vi "Offsets Widget Old.vi"(8 "error in (no error)":errorcluster) -> (0 "error out":errorcluster)   [LabVIEW 2013]
uses:
  Popups/Update Offset Actions.ctl
  lib/Data Access Objects/Metadata/Persistant DAO Actions.ctl
  lib/Data Access Objects/Metadata/DAO Actions.ctl
  lib/Global Data/Dataset Source.ctl
  lib/Global Data/Transactions/Dataset Type.ctl
  lib/Apps/Yes No Button.ctl
  lib/Global Data/Transactions/Dataset Transaction Id.ctl
  lib/Data Access Objects/Metadata/DAO Actions with Remove.ctl
  lib/Launcher/Launcher Actions.ctl
  lib/Launcher/NoPanelAppTypes.ctl
  lib/Offsets/Offset Types.ctl
  Popups/Offset Message.ctl
  <vilib>/Utility/miscctls.llb/LVPointTypeDef.ctl
  lib/Data Display/External Sensor Name Offset & Value.ctl
  lib/Offsets Widget/Offset Widget Actions.ctl
  lib/MixedMode/Messages/MM Widget Parameter Changes.ctl
  lib/Apps/GUI Control.ctl
  Popups/Offset Table Component.ctl
  lib/Offsets Widget/Cartesian Or Actuator.ctl
panel:
  in  "HasBeenModified":bool
  in  "External Sensors Label":string[](array[string])
  in  "External Sensors Table":T1[](array[typedef])
  in  "Table 5":T2 {"Table Data 1" format="%^#_7e"}
  in  "Table 4":T2 {"Table Data 1" format="%^#_7e"}
  in  "Table 3":T2 {"Table Data 1" format="%^#_7e"}
  in  "Table 2":T2 {"Table Data 1" format="%^#_7e"}
  in  "Table 1":T2 {"Table Data 1" format="%^#_7e"}
  in  "Row Labels":string[](array[string])
  in  "Table 0":T2 {"Table Data 1" format="%^#_7e"}
  out "Default Data":dbl[][](array[numeric])
  out "Default Transactions":T3[](array[typedef])
  in  "Coordinate Space":T7 caption="Coord"
  in  "Cartesian Type":bool caption="Coord"
  in  "Force Offset Tag":u16(ring) items=["<None>"]
  in  "Offset Type":T8
  in  "Load":bool
  in  "Number Of Samples":i32
  in  "Sample Interval\n(milliseconds)":dbl
  in  "Offset Widget Actions":T9
  in  "Execute":bool
  in  "Cancel":bool
  in  "Ok":bool
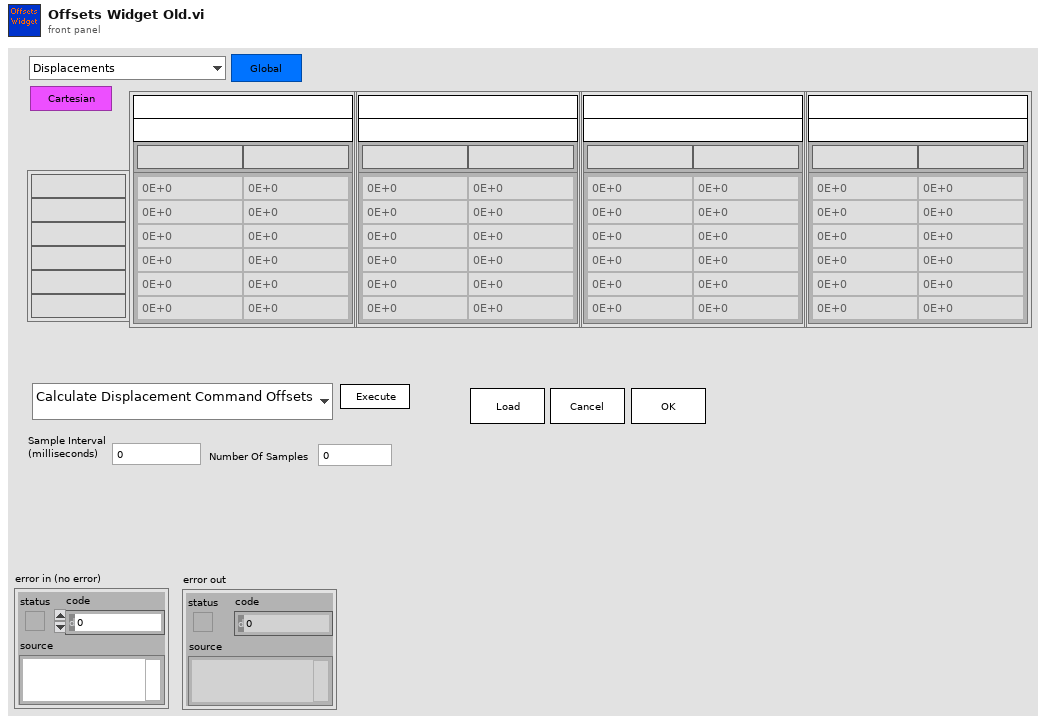
[diagram p1: front panel]
types:
  T1 = typedef "External Sensor Name Offset & Value.ctl" = cluster{"Name":string, "Offset":dbl, "Value 2":dbl}
  T2 = typedef "Offset Table Component.ctl" = cluster{"Table Data 1":dbl[][], "Offset or Current Label":string[], "DOF Label":string, "LBCB Label":string}
  T3 = typedef "Dataset Transaction Id.ctl" = cluster{"Dataset Source":T4, "Dataset Type":T5, "Hold":T6, "Volts":T6, "Tag":string}
  T4 = typedef "Dataset Source.ctl" = enum16{"Continuous", "Hold", "ED", "Volts", "Offsets", "Increments"}
  T5 = typedef "Dataset Type.ctl" = enum16{"LVDT", "Load Cell", "Actuator Command", "Servo Error", "Displacement Command", "Displacement", "Force"}
  T6 = typedef "Yes No Button.ctl" = bool
  T7 = typedef "Cartesian Or Actuator.ctl" = bool
  T8 = typedef "Offset Types.ctl" = enum16{"Displacements", "Forces", "External Sensors"}
  T9 = typedef "Offset Widget Actions.ctl" = enum16{"Calculate Displacement Command Offsets", "Calculate Displacement Offsets", "Calculate Force Offsets", "Calculate External Sensor Offsets"}
  T10 = typedef "GUI Control.ctl" = cluster{"Command":T11, "LBCB Number":enum16{"LBCB1", "LBCB2"}}
  T11 = typedef "MM Widget Parameter Changes.ctl" = enum16{"Start", "Stop All", "Control Enabled", "Control Disabled"}
  T12 = typedef "Offset Message.ctl" = cluster{"Update Offset Actions":T13, "Offset Type":T8, "Coordinate Space":bool, "Cartesian Type":bool}
  T13 = typedef "Update Offset Actions.ctl" = enum16{"Update Table", "Calculate Cartesian Offsets", "Redo Headers", "Has Been Modified", "Exit"}
  T14 = typedef "Persistant DAO Actions.ctl" = enum16{"Init", "Get", "Set", "Load", "Save"}
  T15 = typedef "LVPointTypeDef.ctl" = cluster{"Horizontal":i16, "Vertical":i16}
  T16 = typedef "DAO Actions.ctl" = enum16{"Init", "Get", "Set"}
  T17 = typedef "LVRectTypeDef.ctl" = cluster{"Left":i16, "Top":i16, "Right":i16, "Bottom":i16}
  T18 = typedef "App Parameters.ctl" = cluster{"Monitor Loop":T19, "Ramp Time":T19, "Log Loop":T19, "TCP to DAQ":T19, "Logging Directory":path, "Log File Size (MBytes)":i64, "Volt Logging Loop":T19, "2 LBCB Archiving Mode":bool, "Fake":bool}
  T19 = typedef "Timing Parameters.ctl" = cluster{"Interval":dbl, "Rate ":dbl}
  T20 = typedef "Number Of LBCBs.ctl" = enum16{"1", "2"}
  T21 = cluster{"Table Data 1":dbl[][], "Offset or Current Label":string[], "DOF Label":string, "LBCB Label":string}
  T22 = typedef "DAO Actions with Remove.ctl" = enum16{"Init", "Get", "Set", "Remove"}
  T23 = typedef "NoPanelAppTypes.ctl" = enum16{"NTCP Socket", "Data Archiving", "DAQ Link", "Control Loops", "Cmd Disp Diffs", "LBCB Data", "Limits", "Mixed Mode Widget", "Offsets", "Debug"}
  T24 = typedef "Launcher Actions.ctl" = enum16{"Launch", "Stop All", "Stop", "Kill", "Running?", "Init"}
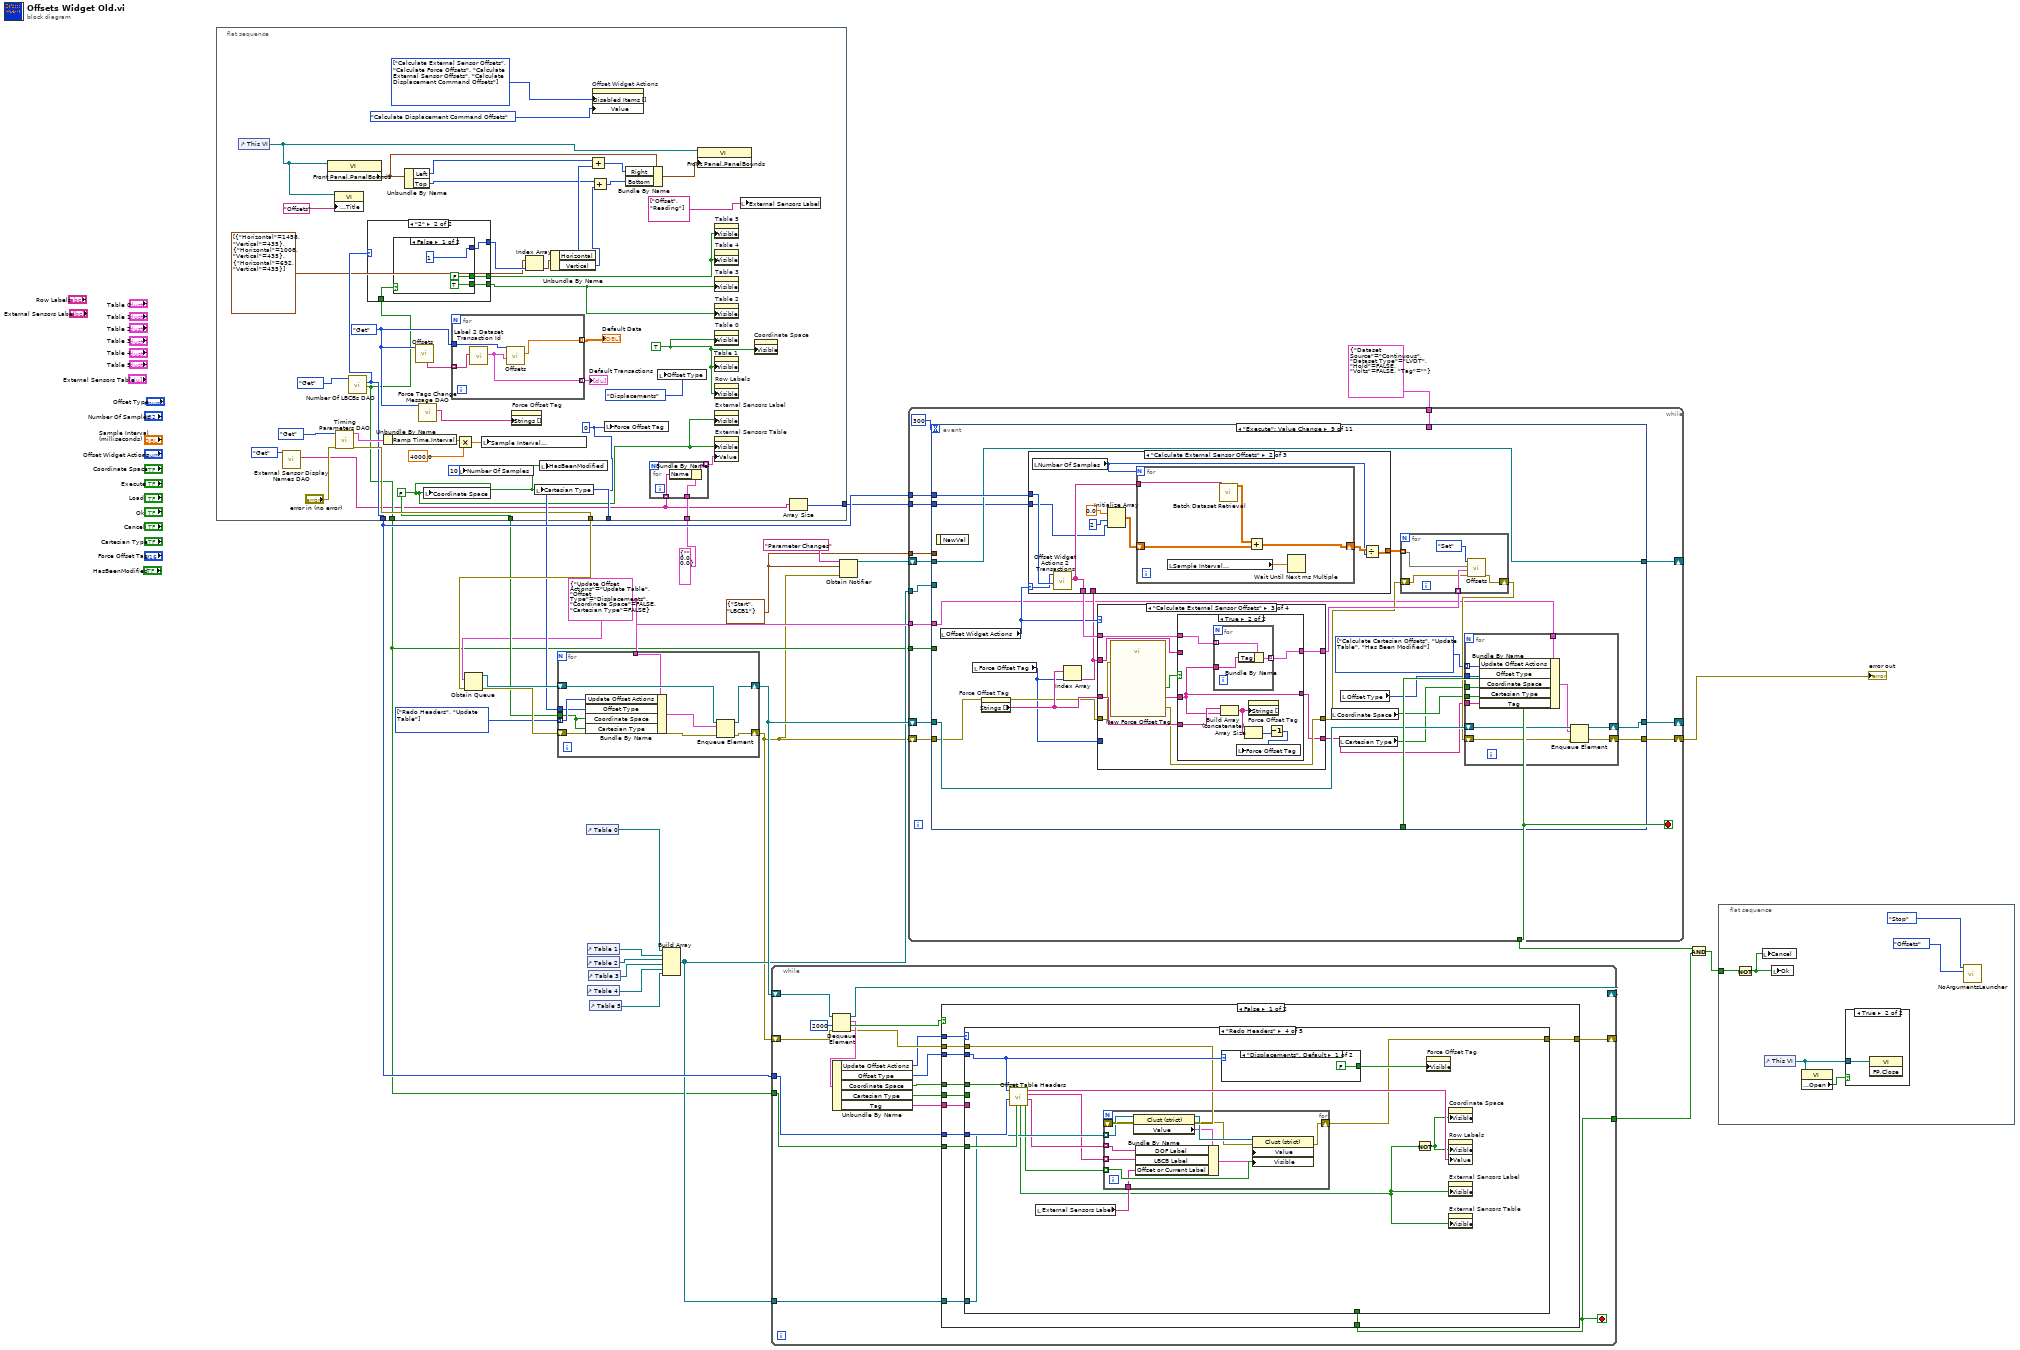
[diagram p0: block diagram]
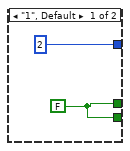
[diagram p2: hidden frame]
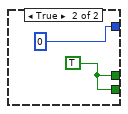
[diagram p3: hidden frame]
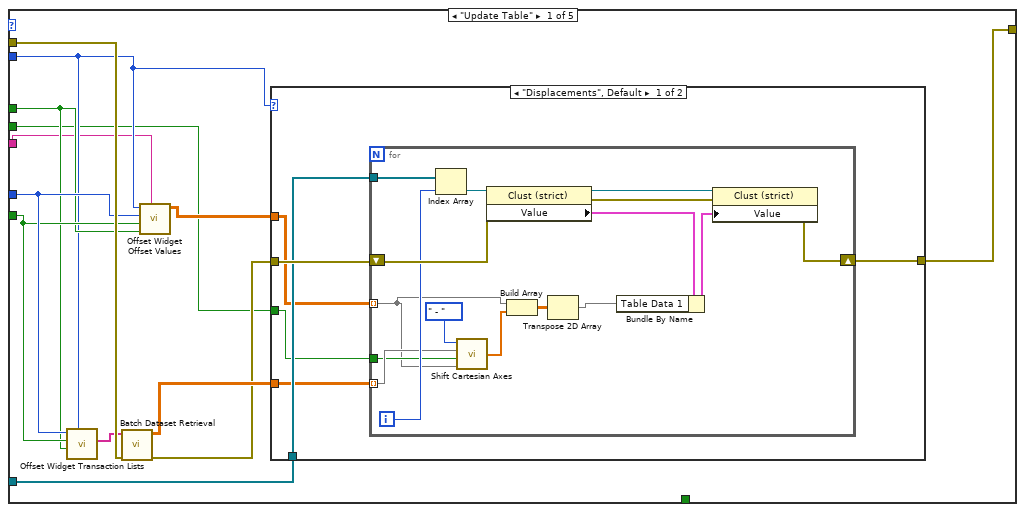
[diagram p5: hidden frame]
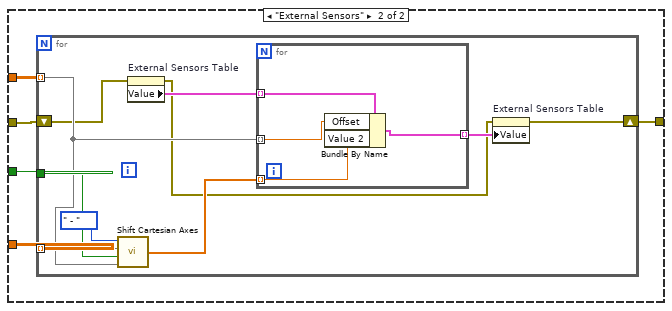
[diagram p6: hidden frame]
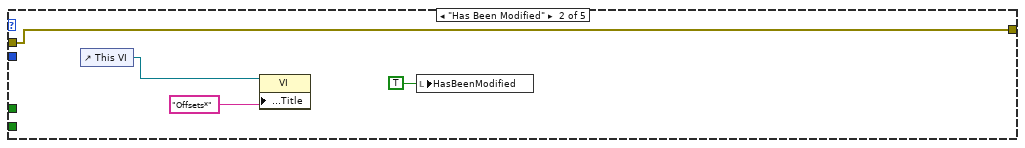
[diagram p7: hidden frame]
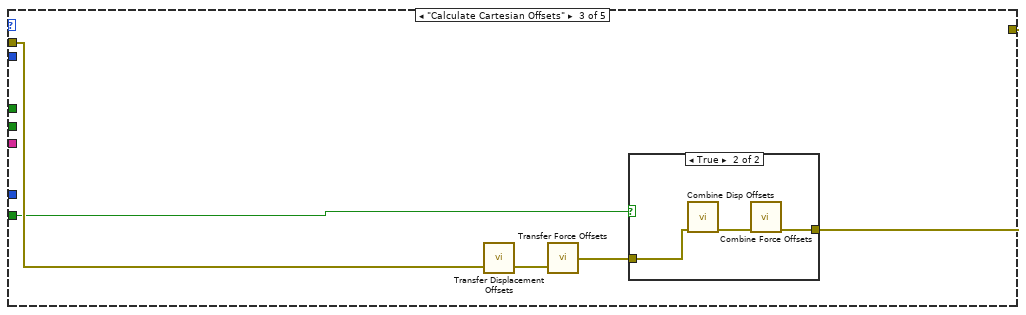
[diagram p8: hidden frame]
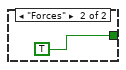
[diagram p10: hidden frame]
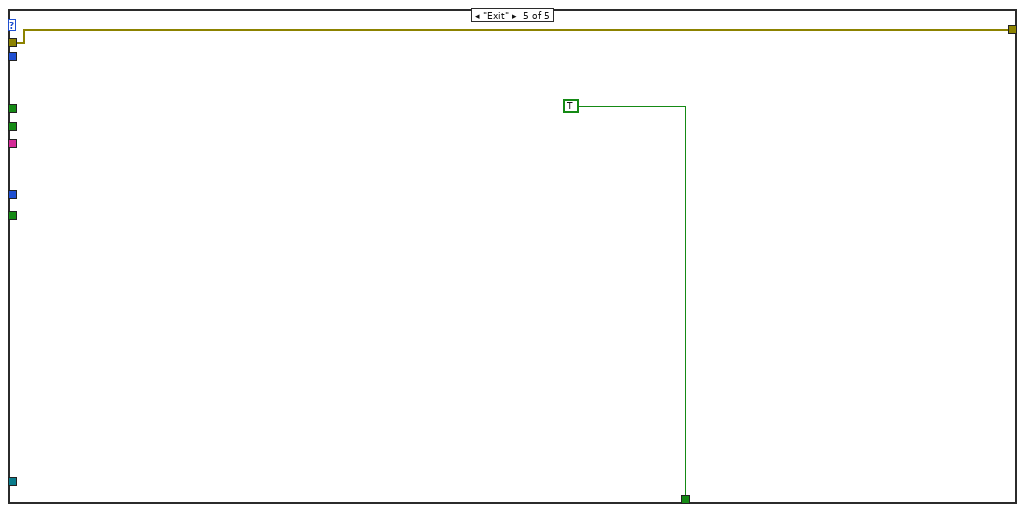
[diagram p11: hidden frame]
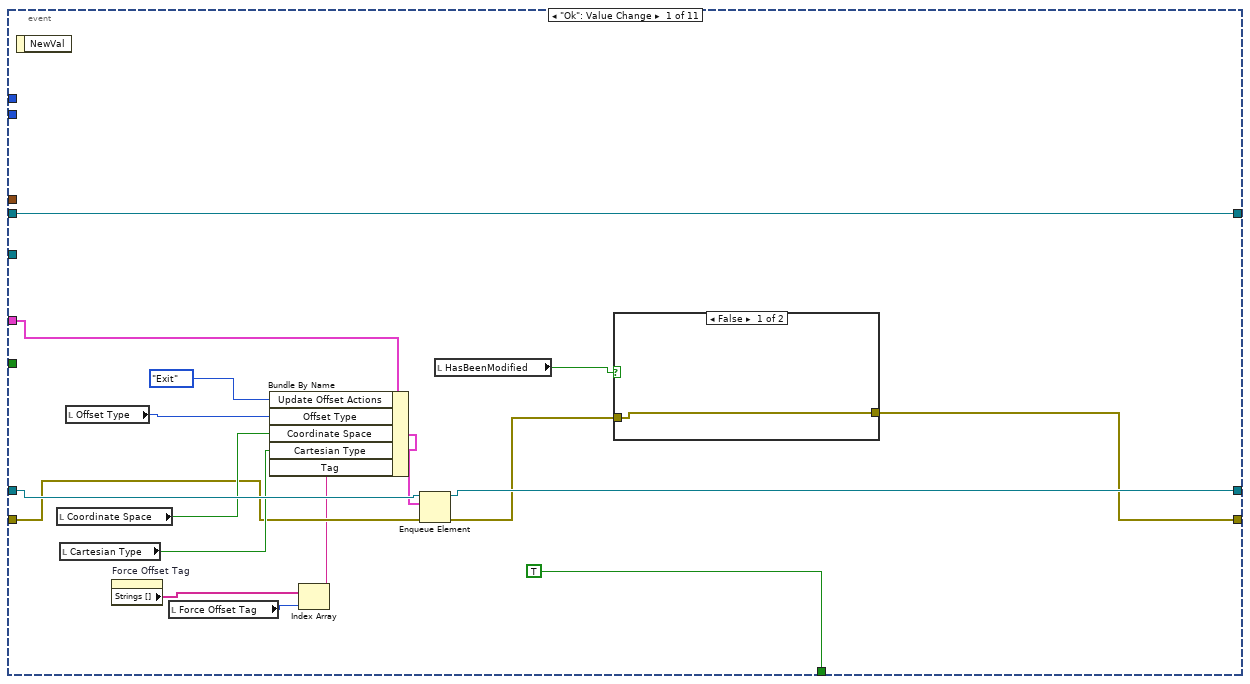
[diagram p13: hidden frame]
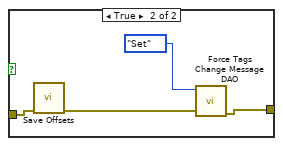
[diagram p14: hidden frame]
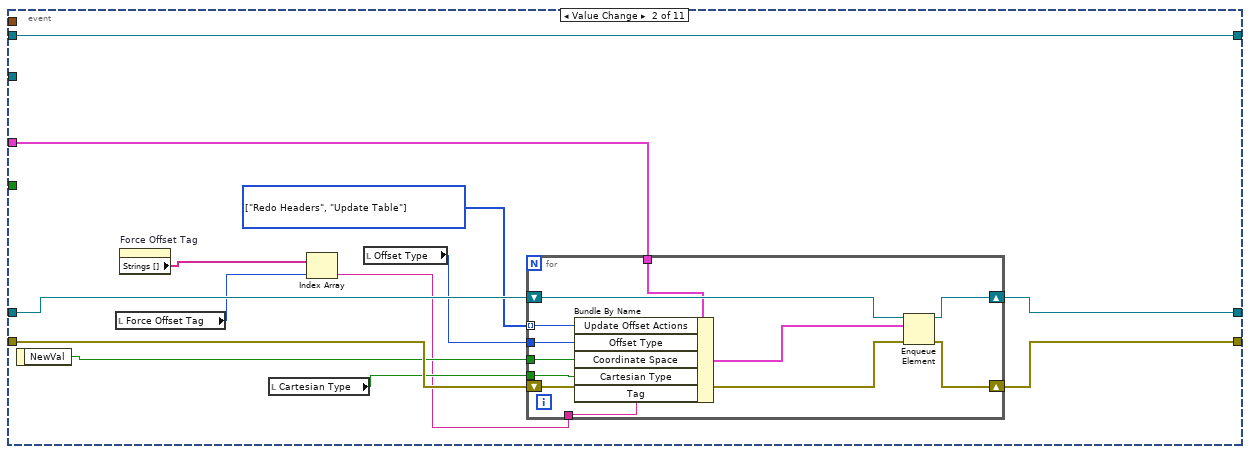
[diagram p15: hidden frame]
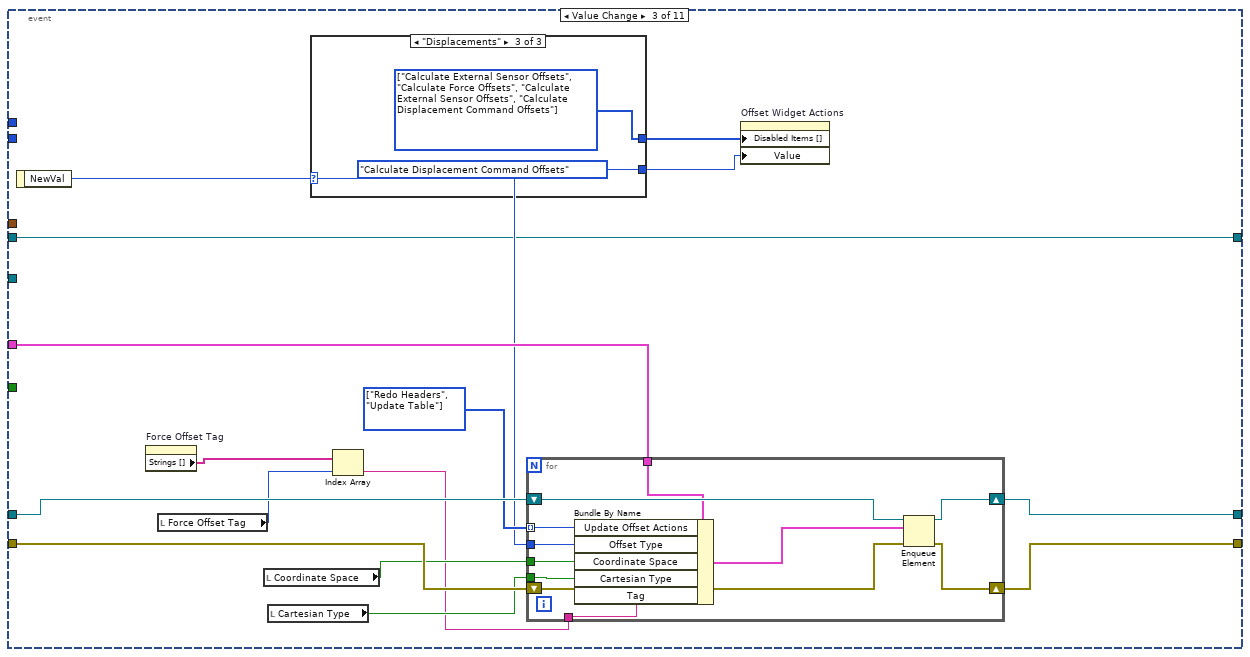
[diagram p16: hidden frame]
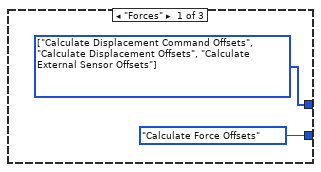
[diagram p17: hidden frame]
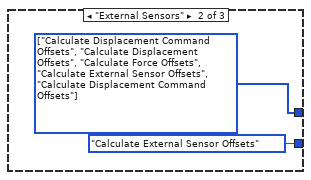
[diagram p18: hidden frame]
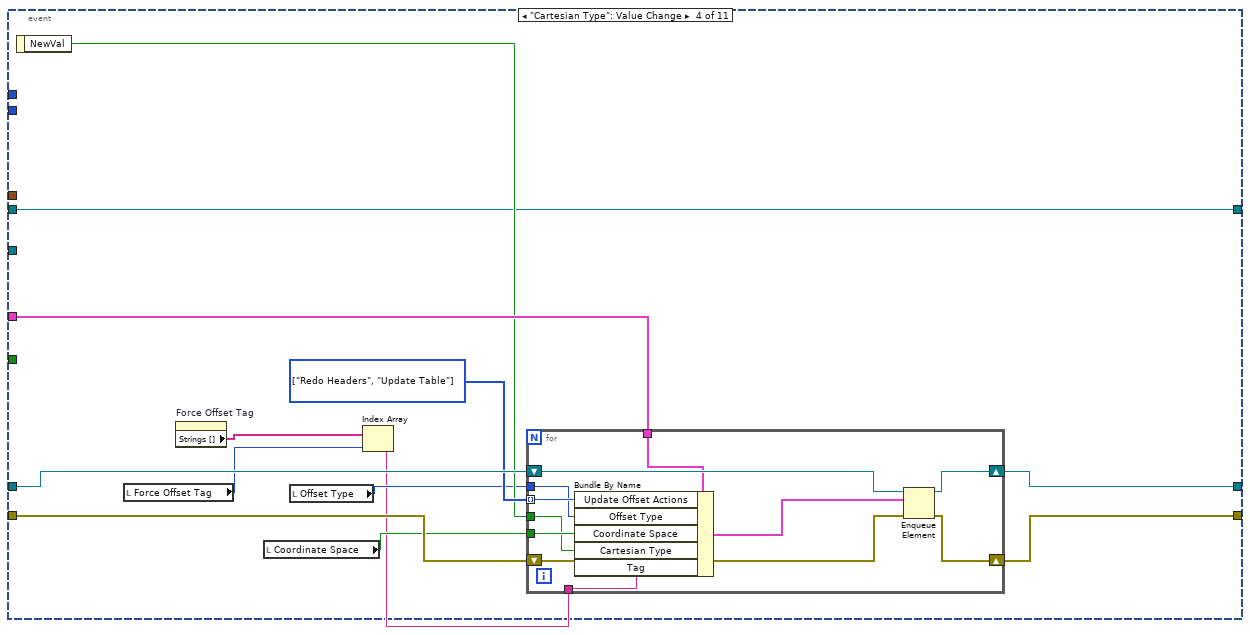
[diagram p19: hidden frame]
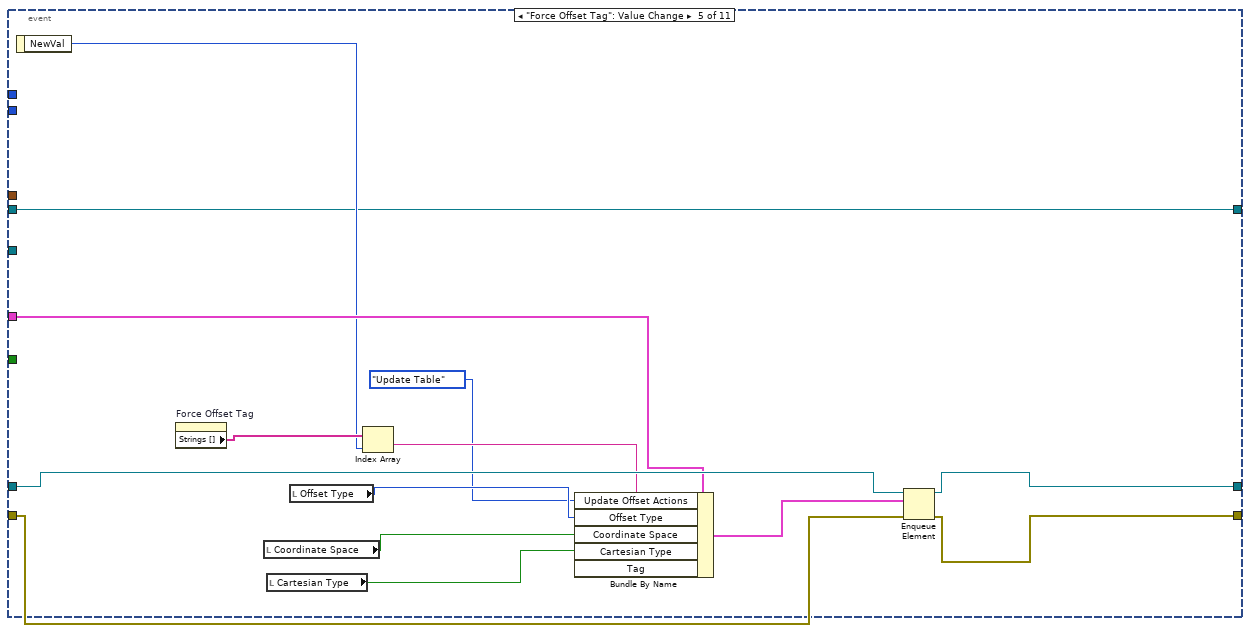
[diagram p20: hidden frame]
diagram:
  w2 = T10 {"Command"=enum."Start", "LBCB Number"=enum."LBCB1"} ("GUI Control")
  w16 = T12 {"Update Offset Actions"=enum."Update Table", "Offset Type"=enum."Displacements", "Coordinate Space"=FALSE, "Cartesian Type"=FALSE} ("Offset Message")
  w19 = T13[] [enum."Redo Headers", enum."Update Table"] items=["Update Table", "Calculate Cartesian Offsets", "Redo Headers", "Has Been Modified", "Exit"]
  n1 = flat-sequence {
    tunnel: [w58] -> w21
    tunnel: [w55] -> w20
    tunnel: [w54] -> w6
    tunnel: [w57] -> w18
    tunnel: [w32] -> w17
    tunnel: T1 {"Name"="", "Offset"=0.0, "Value 2"=0.0} ("External Sensor Name & Value") -> [w47]
    tunnel: [w29] -> w1
    frame #0 {
      w36 = T9[] [enum."Calculate External Sensor Offsets", enum."Calculate Force Offsets", enum."Calculate External Sensor Offsets", enum."Calculate Displacement Command Offsets"] items=["Calculate Displacement Command Offsets", "Calculate Displacement Offsets", "Calculate Force Offsets", "Calculate External Sensor Offsets"] ("Disabled Items []")
      w31 = TRUE ("Visible")
      w32 = FALSE ("Coordinate Space")
      w59 = DAO_Actions."Get" ("DAO Actions")
      w57 = 0
      n2 = control-ref of="This VI"() -> (w34:refnum<vi>)
      n3 = call "External Sensor Display Names DAO.vi"("Persistent DAO Actions"=Persistant_DAO_Actions."Get") -> ("Display Name Out"=w30:string[])  [unwired: 8 in, 2 out]
      n4 = property class="VI"(reference=w34) -> ("Front Panel.PanelBounds"=w41:T17)  [unwired: 1 in, 2 out]
      n5 = property class="VI"(reference=w34, "Front Panel.Title"="Offsets" ("Front Panel Window:Title")) -> ()  [unwired: 1 in, 2 out]
      n6 = call "Timing Parameters DAO.vi"("error in (no error)"="error in (no error)", "Actions"=Persistant_DAO_Actions."Get") -> ("error out"=w58:errorcluster, "Application Timing and Logging Out"=w67:T18)  [unwired: 2 in, 6 out]
      n7 = call "Number Of LBCBs DAO.vi"("Actions"=Persistant_DAO_Actions."Get") -> ("Rigid Connection Out"=w54:bool, "Number of\nLBCBs Out"=w55:T20)  [unwired: 7 in, 2 out]
      n8 = case shown="\"2\"" w55 {
        tunnel: w54 -> [_ w80]
        tunnel: [2 w79] -> w53
        tunnel: [w75 w78] -> w50
        tunnel: [w75 w77] -> w49
        frame "1", Default {
          w75 = FALSE
        }
        frame "2" {
          n9 = case shown="False" w80 {
            tunnel: [1 ("f") 0] -> w79
            tunnel: [FALSE w84] -> w78
            tunnel: [TRUE w84] -> w77
            frame False {
            }
            frame True {
              w84 = TRUE
            }
          }
        }
      }
      n10 = Unbundle By Name(w67) -> ("Ramp Time.Interval"=w68:dbl)
      n11 = Unbundle By Name(w41) -> ("Left"=w45:i16, "Top"=w43:i16)
      n12 = call "Offsets.vi"("DAO Actions"=w59) -> ("Labels"=w64:string[])  [unwired: 8 in, 2 out]
      n13 = call "Force Tags Change Message DAO.vi"("DAO Actions"=w59) -> ("Force Tags"=w60:string[])  [unwired: 8 in, 2 out]
      n14 = local write "Coordinate Space"(w32) -> ()
      n15 = for {
        tunnel: w64 -> [w89] mode=indexing
        tunnel: w59 -> [w88]
        tunnel: [w87] -> w63 mode=indexing
        tunnel: [w86] -> w62 mode=indexing
        n16 = call "Label 2 Dataset Transaction Id.vi"("Label"=w89) -> ("Dataset Trans Id"=w87:T3)  [unwired: 10 in]
        n17 = call "Offsets.vi"("Dataset Trans Id"=w87, "DAO Actions"=w88) -> ("Data Out"=w86:dbl[])  [unwired: 7 in, 2 out]
      }
      "Default Transactions" <- w63
      "Default Data" <- w62
      n18 = Multiply(x=w68, y=4000.0) -> (x*y=w70:dbl)
      n19 = local write "Number Of Samples"(10 ("Number Of Samples")) -> ()
      n20 = local write "Sample Interval\n(milliseconds)"(w70) -> ()
      n21 = property on="Force Offset Tag" class="Ring (strict)"("Strings []"=w60) -> ()  [unwired: 2 in, 2 out]
      n22 = Index Array(array=T15[] [{"Horizontal"=1458, "Vertical"=435}, {"Horizontal"=1008, "Vertical"=435}, {"Horizontal"=692, "Vertical"=435}], index=w53) -> (element=w51:T15)
      n23 = local write "Cartesian Type"(w32) -> ()
      n24 = local write "HasBeenModified"(w32) -> ()
      n25 = Unbundle By Name(w51) -> ("Horizontal"=w44:i16, "Vertical"=w42:i16)
      n26 = Add(x=w45, y=w44) -> (x+y=w39:i16)
      n27 = Add(x=w43, y=w42) -> (x+y=w38:i16)
      n28 = property on="Offset Widget Actions" class="Enum (strict)"("Disabled Items []"=w36, "Value"=Offset_Widget_Actions."Calculate Displacement Command Offsets" ("Offset Widget Actions")) -> ()  [unwired: 2 in, 2 out]
      n29 = local write "Force Offset Tag"(w57) -> ()
      n30 = Bundle By Name(cluster=w41, "Right"=w39, "Bottom"=w38) -> (w40:T17)
      n31 = for {
        tunnel: [w74] -> w48 mode=indexing
        tunnel: w47 -> [w73]
        tunnel: w30 -> [w72] mode=indexing
        n32 = Bundle By Name(cluster=w73, "Name"=w72) -> (w74:T1)
      }
      n33 = local write "Offset Type"(Offset_Types."Displacements" ("Offset Type")) -> ()
      n34 = property class="VI"(reference=w34, "Front Panel.PanelBounds"=w40) -> ()  [unwired: 1 in, 2 out]
      n35 = property on="Table 5" class="Clust (strict)"("Visible"=w50) -> ()  [unwired: 2 in, 2 out]
      n36 = property on="Table 4" class="Clust (strict)"("Visible"=w50) -> ()  [unwired: 2 in, 2 out]
      n37 = property on="Table 3" class="Clust (strict)"("Visible"=w49) -> ()  [unwired: 2 in, 2 out]
      n38 = property on="Table 2" class="Clust (strict)"("Visible"=w49) -> ()  [unwired: 2 in, 2 out]
      n39 = property on="Table 0" class="Clust (strict)"("Visible"=w31) -> ()  [unwired: 2 in, 2 out]
      n40 = property on="Table 1" class="Clust (strict)"("Visible"=w31) -> ()  [unwired: 2 in, 2 out]
      n41 = property on="Row Labels" class="Arr (strict)"("Visible"=w31) -> ()  [unwired: 2 in, 2 out]
      n42 = property on="External Sensors Label" class="Arr (strict)"("Visible"=w32) -> ()  [unwired: 2 in, 2 out]
      n43 = property on="External Sensors Table" class="Arr (strict)"("Visible"=w32, "Value"=w48) -> ()  [unwired: 2 in, 2 out]
      n44 = local write "External Sensors Label"(string[] ["Offset", "Reading"] ("External Sensors Label")) -> ()
      n45 = property on="Coordinate Space" class="Bool (strict)"("Visible"=w31) -> ()  [unwired: 2 in, 2 out]
      n46 = Array Size(array=w30) -> (size(s)=w29:i32)
    }
  }
  n47 = Obtain Queue(element data type=w16, error in (no error)=w21) -> (queue out=w27:refnum<queue>, error out=w28:errorcluster)  [unwired: 3 in, 1 out]
  n48 = for {
    tunnel: w19 -> [w95] mode=indexing
    shift-right: [w96] -> w26
    shift-left: w27 -> [w97]
    shift-right: [w94] -> w3
    shift-left: w28 -> [w98]
    tunnel: w16 -> [w92]
    tunnel: w18 -> [w91]
    tunnel: w17 -> [w90]
    n49 = Bundle By Name(cluster=w92, "Update Offset Actions"=w95, "Offset Type"=w91, "Coordinate Space"=w90, "Cartesian Type"=w90) -> (w93:T12)
    n50 = Enqueue Element(queue=w97, element=w93, error in (no error)=w98) -> (queue out=w96:refnum<queue>, error out=w94:errorcluster)  [unwired: 1 in, 1 out]
  }
  n51 = control-ref of="Table 0"() -> (w15:refnum<vi>)
  n52 = control-ref of="Table 1"() -> (w14:refnum<vi>)
  n53 = control-ref of="Table 2"() -> (w13:refnum<vi>)
  n54 = control-ref of="Table 4"() -> (w11:refnum<vi>)
  n55 = control-ref of="Table 3"() -> (w12:refnum<vi>)
  n56 = control-ref of="Table 5"() -> (w10:refnum<vi>)
  n57 = Build Array(w15, w14, w13, w12, w11, w10) -> (w8:refnum<vi>[])
  n58 = while {
    shift-right: [w112] -> _
    shift-left: w26 -> [w114]
    shift-right: [w108] -> _
    shift-left: w3 -> [w113]
    tunnel: [w107] -> w23
    tunnel: w20 -> [w106]
    tunnel: w6 -> [w105]
    tunnel: w8 -> [w101]
    stop <- w107 stop-if-true
    n59 = Dequeue Element(queue=w114, timeout in ms (-1)=2000, error in (no error)=w113) -> (queue out=w112:refnum<queue>, element=w110:T12, timed out?=w111:bool, error out=w109:errorcluster)
    n60 = Unbundle By Name(w110) -> ("Update Offset Actions"=w104:T13, "Offset Type"=w103:T8, "Coordinate Space"=w102:bool, "Cartesian Type"=w100:bool, "Tag"=w99:string)
    n61 = case shown="False" w111 {
      tunnel: w104 -> [w126 _]
      tunnel: w109 -> [w125 w224]
      tunnel: [w124 w224] -> w108
      tunnel: [w123 _] -> w107
      tunnel: w103 -> [w122 _]
      tunnel: w106 -> [w121 _]
      tunnel: w105 -> [w120 _]
      tunnel: w102 -> [w119 _]
      tunnel: w101 -> [w118 _]
      tunnel: w100 -> [w117 _]
      tunnel: w99 -> [w116 _]
      frame False {
        n62 = case shown="\"Redo Headers\"" w126 {
          tunnel: w125 -> [w139 w181 w186 w197 w222]
          tunnel: [w130 w181 w188 w198 w222] -> w124
          tunnel: [_ _ _ _ TRUE] -> w123
          tunnel: w122 -> [w129 _ _ w207 _]
          tunnel: w121 -> [w136 _ _ w206 _]
          tunnel: w120 -> [w135 _ w185 w204 _]
          tunnel: w119 -> [w134 _ _ w205 _]
          tunnel: w118 -> [w132 _ _ w202 _]
          tunnel: w117 -> [w128 _ _ _ _]
          tunnel: w116 -> [w127 _ _ _ _]
          frame "Update Table" {
            n63 = call "Offset Widget Transaction Lists.vi"("Offset Type"=w129, "Coordinate Space"=w134, "Rigid Connection"=w135, "Number of\nLBCBs"=w136) -> ("Transactions"=w133:string[])  [unwired: 6 in, 1 out]
            n64 = call "Batch Dataset Retrieval.vi"("error in"=w139, "Transactions"=w133) -> ("error out"=w131:errorcluster, "Data"=w138:dbl[][])  [unwired: 8 in]
            n65 = call "Offset Widget Offset Values.vi"(7:w127, "Coordinate Space"=w134, "Rigid Connection In"=w135, "Number of\nLBCBs"=w136, "Offset Type"=w129) -> ("Offsets"=w137:dbl[][])  [unwired: 6 in]
            n66 = case shown="\"Displacements\", Default" w129 {
              tunnel: w138 -> [w142 w166]
              tunnel: w137 -> [w141 w165]
              tunnel: w128 -> [w140 w164]
              tunnel: w132 -> [w143 _]
              tunnel: w131 -> [w145 w163]
              tunnel: [w144 w162] -> w130
              frame "Displacements", Default {
                n67 = for {
                  shift-right: [w159] -> w144
                  shift-left: w145 -> [w161]
                  tunnel: w143 -> [w158]
                  tunnel: w142 -> [w152] mode=indexing
                  tunnel: w141 -> [w150] mode=indexing
                  tunnel: w140 -> [w151]
                  i -> [w157]
                  n68 = Index Array(array=w158, index=w157) -> (element=w156:refnum<vi>)
                  n69 = call "Shift Cartesian Axes.vi"("Coordinate Offset"=w150, "Coordinate Switch"=w151, "Coordinate Input"=w152, "Direction"=enum16{" +", " - "}." - ") -> ("Coordinate Output"=w149:dbl[])
                  n70 = property class="Clust (strict)"(reference=w156, error in=w161) -> (reference out=w155:refnum<vi>, error out=w160:errorcluster, "Value"=w154:T21)
                  n71 = Build Array(w150, w149) -> (w148:dbl[][])
                  n72 = Transpose 2D Array(2D array=w148) -> (transposed array=w147:dbl[][])
                  n73 = Bundle By Name(cluster=w154, "Table Data 1"=w147) -> (w146:T21)
                  n74 = property class="Clust (strict)"(reference=w155, error in=w160, "Value"=w146) -> (error out=w159:errorcluster)  [unwired: 1 out]
                }
              }
              frame "External Sensors" {
                n75 = for {
                  tunnel: w166 -> [w176] mode=indexing
                  tunnel: w164 -> [w175]
                  tunnel: w165 -> [w172] mode=indexing
                  shift-right: [w169] -> w162
                  shift-left: w163 -> [w168]
                  n76 = call "Shift Cartesian Axes.vi"("Coordinate Offset"=w172, "Coordinate Switch"=w175, "Coordinate Input"=w176, "Direction"=enum16{" +", " - "}." - ") -> ("Coordinate Output"=w171:dbl[])
                  n77 = property on="External Sensors Table" class="Arr (strict)"(error in=w168) -> (error out=w167:errorcluster, "Value"=w173:T1[])  [unwired: 1 in, 1 out]
                  n78 = for {
                    tunnel: w173 -> [w180] mode=indexing
                    tunnel: w172 -> [w179] mode=indexing
                    tunnel: w171 -> [w178] mode=indexing
                    tunnel: [w177] -> w170 mode=indexing
                    n79 = Bundle By Name(cluster=w180, "Offset"=w179, "Value 2"=w178) -> (w177:T1)
                  }
                  n80 = property on="External Sensors Table" class="Arr (strict)"(error in=w167, "Value"=w170) -> (error out=w169:errorcluster)  [unwired: 1 in, 1 out]
                }
              }
            }
          }
          frame "Has Been Modified" {
            n81 = control-ref of="This VI"() -> (w184:refnum<vi>)
            n82 = property class="VI"(reference=w184, "Front Panel.Title"="Offsets*" ("Front Panel Window:Title")) -> ()  [unwired: 1 in, 2 out]
            n83 = local write "HasBeenModified"(TRUE ("HasBeenModified")) -> ()
          }
          frame "Calculate Cartesian Offsets" {
            n84 = call "Transfer Displacement Offsets.vi"("error in"=w186) -> ("error out"=w187:errorcluster)  [unwired: 2 in]
            n85 = call "Transfer Force Offsets.vi"("error in"=w187) -> ("error out"=w189:errorcluster)  [unwired: 1 in]
            n86 = case shown="True" w185 {
              tunnel: w189 -> [w190 w193]
              tunnel: [w190 w191] -> w188
              frame False {
              }
              frame True {
                n87 = call "Combine Disp Offsets.vi"("error in (no error)"=w193) -> ("error out"=w192:errorcluster)  [unwired: 10 in]
                n88 = call "Combine Force Offsets.vi"("error in (no error)"=w192) -> ("error out"=w191:errorcluster)  [unwired: 10 in]
              }
            }
          }
          frame "Redo Headers" {
            n89 = call "Offset Table Headers.vi"("Rigid Connection"=w204, "Coordinate Space"=w205, "Number of\nLBCBs"=w206, "Offset Type"=w207) -> ("Visible"=w199:bool[], "Column DOF Headers"=w201:string[], "Column LBCB Headers"=w200:string[], "Row Headers"=w203:string[], "Ext Visible"=w195:bool)  [unwired: 3 in]
            n90 = local read "External Sensors Label"() -> (w196:string[])
            n91 = for {
              tunnel: w202 -> [w214] mode=indexing
              tunnel: w201 -> [w217] mode=indexing
              tunnel: w200 -> [w218] mode=indexing
              tunnel: w199 -> [w219] mode=indexing
              shift-right: [w215] -> w198
              shift-left: w197 -> [w212]
              tunnel: w196 -> [w209]
              n92 = property class="Clust (strict)"(reference=w214, error in=w212) -> (reference out=w213:refnum<vi>, error out=w211:errorcluster, "Value"=w210:T21)
              n93 = Bundle By Name(cluster=w210, "DOF Label"=w217, "LBCB Label"=w218, "Offset or Current Label"=w209) -> (w216:T21)
              n94 = property class="Clust (strict)"(reference=w213, error in=w211, "Value"=w216, "Visible"=w219) -> (error out=w215:errorcluster)  [unwired: 1 out]
            }
            n95 = case shown="\"Displacements\", Default" w207 {
              tunnel: [FALSE TRUE] -> w208
              frame "Displacements", Default {
              }
              frame "Forces" {
              }
            }
            n96 = Not(x=w195) -> (.not. x?=w194:bool)
            n97 = property on="Force Offset Tag" class="Ring (strict)"("Visible"=w208) -> ()  [unwired: 2 in, 2 out]
            n98 = property on="Coordinate Space" class="Bool (strict)"("Visible"=w194) -> ()  [unwired: 2 in, 2 out]
            n99 = property on="Row Labels" class="Arr (strict)"("Visible"=w194, "Value"=w203) -> ()  [unwired: 2 in, 2 out]
            n100 = property on="External Sensors Label" class="Arr (strict)"("Visible"=w195) -> ()  [unwired: 2 in, 2 out]
            n101 = property on="External Sensors Table" class="Arr (strict)"("Visible"=w195) -> ()  [unwired: 2 in, 2 out]
          }
          frame "Exit" {
          }
        }
      }
      frame True {
      }
    }
  }
  n102 = Obtain Notifier(name (unnamed)="Parameter Changes", notification data type=w2, error in (no error)=w3) -> (notifier out=w4:refnum<notifier>)  [unwired: 1 in, 2 out]
  n103 = while {
    shift-right: [w237] -> _
    shift-left: w26 -> [w239]
    shift-right: [w236] -> w25
    shift-left: w3 -> [w238]
    tunnel: [w234] -> w24
    tunnel: w20 -> [w233]
    tunnel: w16 -> [w232]
    tunnel: w8 -> [w231]
    tunnel: T3 {"Dataset Source"=enum."Continuous", "Dataset Type"=enum."LVDT", "Hold"=FALSE, "Volts"=FALSE, "Tag"=""} ("Dataset Trans Id") -> [w230]
    tunnel: w6 -> [w229]
    tunnel: w2 -> [w227]
    shift-right: [w226] -> _
    shift-left: w4 -> [w228]
    tunnel: w1 -> [w225]
    stop <- w234 stop-if-true
    n104 = event shown="[8] \"Execute\": Value Change" {
      selector: _ -> [_ _ _ _ _ _ _ _ _ _ _]
      dyn-events: _ -> [_ _ _ _ _ _ _ _ _ _ _]
      timeout: 300 -> [_ _ _ _ _ _ _ _ _ _ _]
      tunnel: [TRUE _ _ _ _ _ TRUE TRUE _ _ _] -> w234
      tunnel: w239 -> [w255 w274 w300 w330 w355 w361 w408 w425 w449 w567 w661]
      tunnel: w238 -> [w245 w273 w299 w329 w354 w364 w405 w422 w439 w579 w658]
      tunnel: [w254 w271 w297 w327 w352 w360 w407 w424 w447 w568 w660] -> w237
      tunnel: [w243 w272 w298 w328 w353 w357 w406 w423 w448 w569 w659] -> w236
      tunnel: w233 -> [_ _ _ _ _ _ _ _ w446 w573 _]
      tunnel: w232 -> [w252 w269 w295 w325 w351 w359 w401 w418 w435 w564 w656]
      tunnel: w231 -> [_ _ _ _ _ _ _ _ _ w577 _]
      tunnel: w230 -> [_ _ _ _ _ _ _ _ _ w574 _]
      tunnel: w229 -> [_ _ _ _ _ _ _ _ _ w572 _]
      tunnel: w228 -> [w240 w262 w286 w318 w342 w362 w393 w410 w429 w559 w664]
      tunnel: w227 -> [_ _ _ _ _ _ _ _ _ _ _]
      tunnel: [w240 w262 w286 w318 w342 w362 w393 w410 w429 w559 w664] -> w226
      tunnel: w225 -> [_ _ _ _ _ _ _ _ w427 _ _]
      event "Ok": Value Change {
        n105 = event-data() -> ()  [unwired: 2 out]
        n106 = local read "Coordinate Space"() -> (w249:T7)
        n107 = local read "Cartesian Type"() -> (w248:bool)
        n108 = local read "Offset Type"() -> (w250:T8)
        n109 = property on="Force Offset Tag" class="Ring (strict)"() -> ("Strings []"=w247:string[])  [unwired: 2 in, 2 out]
        n110 = local read "Force Offset Tag"() -> (w246:u16)
        n111 = Index Array(array=w247, index=w246) -> (element=w241:string)
        n112 = Bundle By Name(cluster=w252, "Update Offset Actions"=Update_Offset_Actions."Exit" ("notification"), "Offset Type"=w250, "Coordinate Space"=w249, "Cartesian Type"=w248, "Tag"=w241) -> (w253:T12)
        n113 = Enqueue Element(queue=w255, element=w253, error in (no error)=w245) -> (queue out=w254:refnum<queue>, error out=w244:errorcluster)  [unwired: 1 in, 1 out]
        n114 = local read "HasBeenModified"() -> (w242:bool)
        n115 = case shown="False" w242 {
          tunnel: w244 -> [w257 w261]
          tunnel: [w257 w258] -> w243
          frame False {
          }
          frame True {
            n116 = call "Save Offsets.vi"("error in (no error)"=w261) -> ("error out"=w260:errorcluster)  [unwired: 10 out]
            n117 = call "Force Tags Change Message DAO.vi"("error in (no error)"=w260, "DAO Actions"=DAO_Actions."Set") -> ("error out"=w258:errorcluster)  [unwired: 7 in, 2 out]
          }
        }
      }
      event Value Change {
        w270 = T13[] [enum."Redo Headers", enum."Update Table"] items=["Update Table", "Calculate Cartesian Offsets", "Redo Headers", "Has Been Modified", "Exit"]
        n118 = event-data() -> ("NewVal"=w268:T7)  [unwired: 1 out]
        n119 = local read "Force Offset Tag"() -> (w265:u16)
        n120 = property on="Force Offset Tag" class="Ring (strict)"() -> ("Strings []"=w264:string[])  [unwired: 2 in, 2 out]
        n121 = local read "Cartesian Type"() -> (w266:bool)
        n122 = Index Array(array=w264, index=w265) -> (element=w263:string)
        n123 = local read "Offset Type"() -> (w267:T8)
        n124 = for {
          tunnel: w270 -> [w281] mode=indexing
          shift-right: [w282] -> w271
          shift-left: w274 -> [w285]
          shift-right: [w283] -> w272
          shift-left: w273 -> [w284]
          tunnel: w269 -> [w279]
          tunnel: w268 -> [w278]
          tunnel: w267 -> [w277]
          tunnel: w266 -> [w276]
          tunnel: w263 -> [w275]
          n125 = Bundle By Name(cluster=w279, "Update Offset Actions"=w281, "Offset Type"=w277, "Coordinate Space"=w278, "Cartesian Type"=w276, "Tag"=w275) -> (w280:T12)
          n126 = Enqueue Element(queue=w285, element=w280, error in (no error)=w284) -> (queue out=w282:refnum<queue>, error out=w283:errorcluster)  [unwired: 1 in, 1 out]
        }
      }
      event Value Change {
        w296 = T13[] [enum."Redo Headers", enum."Update Table"] items=["Update Table", "Calculate Cartesian Offsets", "Redo Headers", "Has Been Modified", "Exit"]
        n127 = event-data() -> ("NewVal"=w292:T8)  [unwired: 1 out]
        n128 = property on="Force Offset Tag" class="Ring (strict)"() -> ("Strings []"=w288:string[])  [unwired: 2 in, 2 out]
        n129 = local read "Force Offset Tag"() -> (w289:u16)
        n130 = local read "Coordinate Space"() -> (w294:T7)
        n131 = local read "Cartesian Type"() -> (w293:bool)
        n132 = case shown="\"Displacements\"" w292 {
          tunnel: [w302 w304 w306] -> w291
          tunnel: [Offset_Widget_Actions."Calculate Force Offsets" ("Offset Widget Actions") Offset_Widget_Actions."Calculate External Sensor Offsets" ("Offset Widget Actions") Offset_Widget_Actions."Calculate Displacement Command Offsets" ("Offset Widget Actions")] -> w290
          frame "Forces" {
            w302 = T9[] [enum."Calculate Displacement Command Offsets", enum."Calculate Displacement Offsets", enum."Calculate External Sensor Offsets"] items=["Calculate Displacement Command Offsets", "Calculate Displacement Offsets", "Calculate Force Offsets", "Calculate External Sensor Offsets"] ("Disabled Items []")
          }
          frame "External Sensors" {
            w304 = T9[] [enum."Calculate Displacement Command Offsets", enum."Calculate Displacement Offsets", enum."Calculate Force Offsets", enum."Calculate External Sensor Offsets", enum."Calculate Displacement Command Offsets"] items=["Calculate Displacement Command Offsets", "Calculate Displacement Offsets", "Calculate Force Offsets", "Calculate External Sensor Offsets"] ("Disabled Items []")
          }
          frame "Displacements" {
            w306 = T9[] [enum."Calculate External Sensor Offsets", enum."Calculate Force Offsets", enum."Calculate External Sensor Offsets", enum."Calculate Displacement Command Offsets"] items=["Calculate Displacement Command Offsets", "Calculate Displacement Offsets", "Calculate Force Offsets", "Calculate External Sensor Offsets"] ("Disabled Items []")
          }
        }
        n133 = Index Array(array=w288, index=w289) -> (element=w287:string)
        n134 = for {
          tunnel: w296 -> [w313] mode=indexing
          shift-right: [w314] -> w297
          shift-left: w300 -> [w317]
          shift-right: [w315] -> w298
          shift-left: w299 -> [w316]
          tunnel: w295 -> [w311]
          tunnel: w294 -> [w310]
          tunnel: w292 -> [w309]
          tunnel: w293 -> [w308]
          tunnel: w287 -> [w307]
          n135 = Bundle By Name(cluster=w311, "Update Offset Actions"=w313, "Offset Type"=w309, "Coordinate Space"=w310, "Cartesian Type"=w308, "Tag"=w307) -> (w312:T12)
          n136 = Enqueue Element(queue=w317, element=w312, error in (no error)=w316) -> (queue out=w314:refnum<queue>, error out=w315:errorcluster)  [unwired: 1 in, 1 out]
        }
        n137 = property on="Offset Widget Actions" class="Enum (strict)"("Disabled Items []"=w291, "Value"=w290) -> ()  [unwired: 2 in, 2 out]
      }
      event "Cartesian Type": Value Change {
        w326 = T13[] [enum."Redo Headers", enum."Update Table"] items=["Update Table", "Calculate Cartesian Offsets", "Redo Headers", "Has Been Modified", "Exit"]
        n138 = event-data() -> ("NewVal"=w323:bool)  [unwired: 1 out]
        n139 = local read "Force Offset Tag"() -> (w321:u16)
        n140 = property on="Force Offset Tag" class="Ring (strict)"() -> ("Strings []"=w320:string[])  [unwired: 2 in, 2 out]
        n141 = local read "Coordinate Space"() -> (w324:T7)
        n142 = local read "Offset Type"() -> (w322:T8)
        n143 = Index Array(array=w320, index=w321) -> (element=w319:string)
        n144 = for {
          tunnel: w326 -> [w337] mode=indexing
          shift-right: [w338] -> w327
          shift-left: w330 -> [w341]
          shift-right: [w339] -> w328
          shift-left: w329 -> [w340]
          tunnel: w325 -> [w335]
          tunnel: w324 -> [w334]
          tunnel: w323 -> [w333]
          tunnel: w322 -> [w332]
          tunnel: w319 -> [w331]
          n145 = Bundle By Name(cluster=w335, "Update Offset Actions"=w337, "Offset Type"=w332, "Coordinate Space"=w334, "Cartesian Type"=w333, "Tag"=w331) -> (w336:T12)
          n146 = Enqueue Element(queue=w341, element=w336, error in (no error)=w340) -> (queue out=w338:refnum<queue>, error out=w339:errorcluster)  [unwired: 1 in, 1 out]
        }
      }
      event "Force Offset Tag": Value Change {
        n147 = event-data() -> ("NewVal"=w346:u16)  [unwired: 1 out]
        n148 = property on="Force Offset Tag" class="Ring (strict)"() -> ("Strings []"=w348:string[])  [unwired: 2 in, 2 out]
        n149 = local read "Coordinate Space"() -> (w350:T7)
        n150 = local read "Cartesian Type"() -> (w345:bool)
        n151 = local read "Offset Type"() -> (w349:T8)
        n152 = Index Array(array=w348, index=w346) -> (element=w347:string)
        n153 = Bundle By Name(cluster=w351, "Update Offset Actions"=Update_Offset_Actions."Update Table" ("element"), "Offset Type"=w349, "Coordinate Space"=w350, "Cartesian Type"=w345, "Tag"=w347) -> (w343:T12)
        n154 = Enqueue Element(queue=w355, element=w343, error in (no error)=w354) -> (queue out=w352:refnum<queue>, error out=w353:errorcluster)  [unwired: 1 in, 1 out]
      }
      event "Load": Mouse Down? {
        n155 = event-data() -> ()  [unwired: 3 out]
        n156 = local read "Offset Type"() -> (w358:T8)
        n157 = call "Load Offsets.vi"("error in (no error)"=w364) -> ("error out"=w356:errorcluster)  [unwired: 10 in]
        n158 = case shown="No Error" w356 {
          selector: w356 -> [w375 w391]
          tunnel: w361 -> [w378 w392]
          tunnel: [w366 w392] -> w360
          tunnel: w359 -> [w377 _]
          tunnel: w358 -> [w376 _]
          tunnel: [w365 w390] -> w357
          frame No Error {
            w367 = T13[] [enum."Calculate Cartesian Offsets", enum."Update Table"] items=["Update Table", "Calculate Cartesian Offsets", "Redo Headers", "Has Been Modified", "Exit"]
            w368 = u16 0 items=["<None>"] ("Force Offset Tag")
            n159 = local read "Coordinate Space"() -> (w374:T7)
            n160 = local read "Cartesian Type"() -> (w373:bool)
            n161 = call "Force Tags Change Message DAO.vi"("error in (no error)"=w375, "DAO Actions"=DAO_Actions."Get") -> ("error out"=w371:errorcluster, "Force Tags"=w370:string[])  [unwired: 7 in, 1 out]
            n162 = property on="Force Offset Tag" class="Ring (strict)"("Strings []"=w370) -> ()  [unwired: 2 in, 2 out]
            n163 = Index Array(array=w370, index=w368) -> (element=w372:string)
            n164 = local write "Force Offset Tag"(w368) -> ()
            n165 = for {
              tunnel: w377 -> [w384]
              tunnel: w376 -> [w383]
              tunnel: w374 -> [w382]
              tunnel: w373 -> [w381]
              tunnel: w372 -> [w380]
              tunnel: w367 -> [w379] mode=indexing
              shift-right: [w387] -> w366
              shift-left: w378 -> [w388]
              shift-right: [w386] -> w365
              shift-left: w371 -> [w389]
              n166 = Bundle By Name(cluster=w384, "Update Offset Actions"=w379, "Offset Type"=w383, "Coordinate Space"=w382, "Cartesian Type"=w381, "Tag"=w380) -> (w385:T12)
              n167 = Enqueue Element(queue=w388, element=w385, error in (no error)=w389) -> (queue out=w387:refnum<queue>, error out=w386:errorcluster)  [unwired: 1 in, 1 out]
            }
          }
          frame Error {
            n168 = call <vilib>:"Clear Errors.vi"("error in (no error)"=w391) -> ("error out"=w390:errorcluster)  [unwired: 6 in]
          }
        }
        n169 = event-data("Discard?"=TRUE) -> ()  [unwired: 4 in, 1 out]
      }
      event "Cancel": Value Change {
        n170 = event-data() -> ()  [unwired: 2 out]
        n171 = local read "Coordinate Space"() -> (w398:T7)
        n172 = local read "Force Offset Tag"() -> (w395:u16)
        n173 = local read "Offset Type"() -> (w399:T8)
        n174 = local read "Cartesian Type"() -> (w397:bool)
        n175 = property on="Force Offset Tag" class="Ring (strict)"() -> ("Strings []"=w396:string[])  [unwired: 2 in, 2 out]
        n176 = Index Array(array=w396, index=w395) -> (element=w394:string)
        n177 = Bundle By Name(cluster=w401, "Update Offset Actions"=Update_Offset_Actions."Exit" ("notification"), "Offset Type"=w399, "Coordinate Space"=w398, "Cartesian Type"=w397, "Tag"=w394) -> (w400:T12)
        n178 = Enqueue Element(queue=w408, element=w400, error in (no error)=w405) -> (queue out=w407:refnum<queue>, error out=w406:errorcluster)  [unwired: 1 in, 1 out]
        n179 = local read "Default Data"() -> (w403:dbl[][])
        n180 = local read "Default Transactions"() -> (w404:T3[])
        n181 = call "Batch Dataset Store.vi"("Data"=w403, "Transactions"=w404) -> ()  [unwired: 9 in, 1 out]
      }
      event Application Instance Close; Panel Close {
        n182 = event-data() -> ()  [unwired: 2 out]
        n183 = local read "Coordinate Space"() -> (w415:T7)
        n184 = local read "Force Offset Tag"() -> (w411:u16)
        n185 = local read "Cartesian Type"() -> (w414:bool)
        n186 = local read "Offset Type"() -> (w416:T8)
        n187 = property on="Force Offset Tag" class="Ring (strict)"() -> ("Strings []"=w413:string[])  [unwired: 2 in, 2 out]
        n188 = Index Array(array=w413, index=w411) -> (element=w412:string)
        n189 = Bundle By Name(cluster=w418, "Update Offset Actions"=Update_Offset_Actions."Exit" ("notification"), "Offset Type"=w416, "Coordinate Space"=w415, "Cartesian Type"=w414, "Tag"=w412) -> (w419:T12)
        n190 = local read "Default Data"() -> (w420:dbl[][])
        n191 = Enqueue Element(queue=w425, element=w419, error in (no error)=w422) -> (queue out=w424:refnum<queue>, error out=w423:errorcluster)  [unwired: 1 in, 1 out]
        n192 = local read "Default Transactions"() -> (w421:T3[])
        n193 = call "Batch Dataset Store.vi"("Data"=w420, "Transactions"=w421) -> ()  [unwired: 9 in, 1 out]
      }
      event "Execute": Value Change {
        w431 = T13[] [enum."Calculate Cartesian Offsets", enum."Update Table", enum."Has Been Modified"] items=["Update Table", "Calculate Cartesian Offsets", "Redo Headers", "Has Been Modified", "Exit"]
        n194 = event-data() -> ()  [unwired: 2 out]
        n195 = local read "Offset Widget Actions"() -> (w437:T9)
        n196 = local read "Force Offset Tag"() -> (w430:u16)
        n197 = property on="Force Offset Tag" class="Ring (strict)"(error in=w439) -> (error out=w438:errorcluster, "Strings []"=w441:string[])  [unwired: 1 in, 1 out]
        n198 = Index Array(array=w441, index=w430) -> (element=w436:string)
        n199 = case shown="\"Calculate External Sensor Offsets\"" w437 {
          selector: w437 -> [w461 w477 _]
          tunnel: w446 -> [w469 w484 _]
          tunnel: [w468 w483 dbl[][] []] -> w445
          tunnel: [w467 w482 w493] -> w443
          tunnel: w436 -> [_ _ w494]
          tunnel: w427 -> [_ w476 _]
          frame "Calculate Displacement Offsets", Default {
            n200 = local read "Number Of Samples"() -> (w462:i32)
            n201 = call "Offset Widget Actions 2 Transactions.vi"("Number of LBCBs"=w469, "Offset Widget Actions"=w461) -> ("Transactions"=w467:string[])  [unwired: 9 in]
            n202 = Initialize Array(0.0 ("element"), 2 ("dimension size"), 6 ("dimension size")) -> (w463:dbl[][])
            n203 = for {
              N: w462 -> [_]
              shift-right: [w473] -> w470
              shift-left: w463 -> [w475]
              tunnel: w467 -> [w472]
              n204 = local read "Sample Interval\n(milliseconds)"() -> (w474:dbl)
              n205 = call "Batch Dataset Retrieval.vi"("Transactions"=w472) -> ("Data"=w471:dbl[][])  [unwired: 9 in, 1 out]
              n206 = Add(x=w471, y=w475) -> (x+y=w473:dbl[][])
              n207 = Wait Until Next ms Multiple(millisecond multiple=w474) -> ()  [unwired: 1 out]
            }
            n208 = Divide(x=w470, y=w462) -> (x/y=w468:dbl[][])
          }
          frame "Calculate External Sensor Offsets" {
            n209 = local read "Number Of Samples"() -> (w478:i32)
            n210 = call "Offset Widget Actions 2 Transactions.vi"("Number of LBCBs"=w484, "Offset Widget Actions"=w477) -> ("Transactions"=w482:string[])  [unwired: 9 in]
            n211 = Initialize Array(0.0 ("element"), 2 ("dimension size"), w476) -> (w479:dbl[][])
            n212 = for {
              N: w478 -> [_]
              shift-right: [w488] -> w485
              shift-left: w479 -> [w490]
              tunnel: w482 -> [w487]
              n213 = local read "Sample Interval\n(milliseconds)"() -> (w489:dbl)
              n214 = call "Batch Dataset Retrieval.vi"("Transactions"=w487) -> ("Data"=w486:dbl[][])  [unwired: 9 in, 1 out]
              n215 = Add(x=w486, y=w490) -> (x+y=w488:dbl[][])
              n216 = Wait Until Next ms Multiple(millisecond multiple=w489) -> ()  [unwired: 1 out]
            }
            n217 = Divide(x=w485, y=w478) -> (x/y=w483:dbl[][])
          }
          frame "Calculate Displacement Command Offsets" {
            n218 = call "Offsets.vi"("DAO Actions"=DAO_Actions."Get") -> ("Labels"=w495:string[])  [unwired: 8 in, 2 out]
            n219 = for {
              tunnel: w495 -> [w503] mode=indexing
              tunnel: w494 -> [w502]
              shift-right: [w498] -> w493
              shift-left: T3[] [] -> [w497]
              n220 = call "Label 2 Dataset Transaction Id.vi"("Label"=w503) -> ("Dataset Trans Id"=w499:T3)  [unwired: 10 in]
              n221 = Unbundle By Name(w499) -> ("Tag"=w500:string)
              n222 = Equal?(x=w500, y=w502) -> (x = y?=w501:bool)
              n223 = case shown="True" w501 {
                tunnel: w499 -> [_ w507]
                tunnel: [w504 w506] -> w498
                tunnel: w497 -> [w504 w505]
                frame False {
                }
                frame True {
                  n224 = Build Array (concatenate)(w505, w507) -> (w506:T3[])
                }
              }
            }
          }
        }
        n225 = case shown="\"Calculate External Sensor Offsets\"" w437 {
          tunnel: w443 -> [w510 w514 w526 w550]
          tunnel: w436 -> [w508 w511 w518 _]
          tunnel: [w510 w513 w525 T3[] [] ("Transactions")] -> w442
          tunnel: w441 -> [_ _ w524 w545]
          tunnel: w438 -> [w509 w512 w522 w541]
          tunnel: [w509 w512 w521 w540] -> w440
          tunnel: w430 -> [_ _ _ w544]
          tunnel: [w508 w511 w519 w542] -> w428
          frame "Calculate Displacement Offsets", Default {
          }
          frame "Calculate Force Offsets" {
            n226 = for {
              tunnel: w514 -> [w517] mode=indexing
              tunnel: w511 -> [w516]
              tunnel: [w515] -> w513 mode=indexing
              n227 = Bundle By Name(cluster=w517, "Tag"=w516) -> (w515:T3)
            }
          }
          frame "Calculate External Sensor Offsets" {
            n228 = call "New Force Offset Tag"("error in (no error)"=w522) -> ("Force Offset Tag"=w523:string, "OK"=w520:bool, "error out"=w521:errorcluster)  [unwired: 16 in]
            n229 = case shown="True" w520 {
              tunnel: w526 -> [w528 w535]
              tunnel: [w528 w534] -> w525
              tunnel: w524 -> [_ w533]
              tunnel: w523 -> [_ w529]
              tunnel: [w527 w529] -> w519
              tunnel: w518 -> [w527 _]
              frame False {
              }
              frame True {
                n230 = for {
                  tunnel: w535 -> [w538] mode=indexing
                  tunnel: w529 -> [w537]
                  tunnel: [w536] -> w534 mode=indexing
                  n231 = Bundle By Name(cluster=w538, "Tag"=w537) -> (w536:T3)
                }
                n232 = Build Array (concatenate)(w533, w529) -> (w532:string[])
                n233 = Array Size(array=w532) -> (size(s)=w531:i32)
                n234 = property on="Force Offset Tag" class="Ring (strict)"("Strings []"=w532) -> ()  [unwired: 2 in, 2 out]
                n235 = Decrement(x=w531) -> (x-1=w530:i32)
                n236 = local write "Force Offset Tag"(w530) -> ()
              }
            }
          }
          frame "Calculate Displacement Command Offsets" {
            n237 = Decrement(x=w544) -> (x-1=w548:u16)
            n238 = for {
              tunnel: w550 -> [w553] mode=indexing
              n239 = call "Offsets.vi"("Dataset Trans Id"=w553, "DAO Actions"=DAO_Actions_with_Remove."Remove") -> ()  [unwired: 7 in, 3 out]
            }
            n240 = Delete From Array(array=w545, length=1, index=w544) -> (array with subset deleted=w539:string[])  [unwired: 1 out]
            n241 = Less Than 0?(x=w548) -> (x < 0?=w549:bool)
            n242 = Select(t=0, s=w549, f=w548) -> (s? t:f=w546:i32)
            n243 = local write "Force Offset Tag"(w546) -> ()
            n244 = property on="Force Offset Tag" class="Ring (strict)"(error in=w541, "Strings []"=w539) -> (error out=w540:errorcluster)  [unwired: 1 in, 1 out]
            n245 = Index Array(array=w539, index=w546) -> (element=w542:string)
          }
        }
        n246 = local read "Coordinate Space"() -> (w434:T7)
        n247 = local read "Cartesian Type"() -> (w432:bool)
        n248 = local read "Offset Type"() -> (w433:T8)
        n249 = for {
          tunnel: w442 -> [w557] mode=indexing
          tunnel: w445 -> [w556] mode=indexing
          shift-right: [w554] -> w444
          shift-left: w440 -> [w555]
          n250 = call "Offsets.vi"("error in (no error)"=w555, "Dataset Trans Id"=w557, "Data In"=w556, "DAO Actions"=DAO_Actions."Set") -> ("error out"=w554:errorcluster)  [unwired: 5 in, 2 out]
        }
        n251 = for {
          tunnel: w435 -> [w455]
          tunnel: w431 -> [w454] mode=indexing
          tunnel: w434 -> [w453]
          tunnel: w433 -> [w452]
          tunnel: w432 -> [w451]
          shift-right: [w458] -> w447
          shift-left: w449 -> [w460]
          shift-right: [w459] -> w448
          shift-left: w444 -> [w457]
          tunnel: w428 -> [w450]
          n252 = Bundle By Name(cluster=w455, "Update Offset Actions"=w454, "Offset Type"=w452, "Coordinate Space"=w453, "Cartesian Type"=w451, "Tag"=w450) -> (w456:T12)
          n253 = Enqueue Element(queue=w460, element=w456, error in (no error)=w457) -> (queue out=w458:refnum<queue>, error out=w459:errorcluster)  [unwired: 1 in, 1 out]
        }
      }
      event "Table 0", "Table 1", "Table 2", "Table 3", "Table 4", "Table 5": Value Change {
        w566 = T13[] [enum."Calculate Cartesian Offsets", enum."Update Table", enum."Has Been Modified"] items=["Update Table", "Calculate Cartesian Offsets", "Redo Headers", "Has Been Modified", "Exit"]
        n254 = event-data() -> ("CtlRef"=w580:refnum<vi>, "OldVal"=w576:T2, "NewVal"=w575:T2)  [unwired: 1 out]
        n255 = local read "Force Offset Tag"() -> (w561:u16)
        n256 = local read "Coordinate Space"() -> (w565:T7)
        n257 = Search 1D Array(1D array=w577, element=w580) -> (index of element=w578:i32)  [unwired: 1 in]
        n258 = local read "Offset Type"() -> (w563:T8)
        n259 = property on="Force Offset Tag" class="Ring (strict)"() -> ("Strings []"=w571:string[])  [unwired: 2 in, 2 out]
        n260 = Index Array(array=w571, index=w561) -> (element=w560:string)
        n261 = case shown="\"Forces\", Default" w563 {
          tunnel: w579 -> [w593 w627]
          tunnel: [w592 w626] -> w570
          tunnel: w578 -> [w597 w629]
          tunnel: w577 -> [_ w630]
          tunnel: w576 -> [_ w628]
          tunnel: w565 -> [w602 w625]
          tunnel: w575 -> [w601 w622]
          tunnel: w574 -> [w596 w623]
          tunnel: w573 -> [w595 w624]
          tunnel: w572 -> [w594 _]
          tunnel: w560 -> [_ w621]
          frame "Displacements" {
            n262 = Unbundle By Name(w601) -> ("Table Data 1"=w600:dbl[][])
            n263 = Index Array(array=w600, index (col)=0 ("disabled index (col)")) -> (element=w598:dbl[])  [unwired: 1 in]
            n264 = case shown="True" w602 {
              tunnel: w598 -> [w608 w616]
              tunnel: w597 -> [w606 w619]
              tunnel: w596 -> [_ w614]
              tunnel: w595 -> [w607 w613]
              tunnel: w594 -> [w605 _]
              tunnel: w593 -> [w610 w612]
              tunnel: [w609 w611] -> w592
              frame False {
                n265 = call "Table Number 2 Dataset Source.vi"("Rigid Connection"=w605, "Table Number"=w606, "Number of\nLBCBs"=w607) -> ("Dataset Source"=w604:T4, "IsCommand"=w603:bool)  [unwired: 1 in, 1 out]
                n266 = call "Manual Cartesian Displacement Offset.vi"("error in"=w610, "Cartesian Displacements"=w608, "Dataset Source"=w604, "Is Command"=w603) -> ("error out"=w609:errorcluster)  [unwired: 7 in]
              }
              frame True {
                n267 = call "Displacement Table Number 2 Dataset Id.vi"("Table Number"=w619, "Number of\nLBCBs"=w613) -> ("Dataset Source"=w618:T4, "Dataset Type"=w617:T5)  [unwired: 2 in]
                n268 = Bundle By Name(cluster=w614, "Dataset Type"=w617, "Dataset Source"=w618) -> (w615:T3)
                n269 = call "Offsets.vi"("error in (no error)"=w612, "Dataset Trans Id"=w615, "Data In"=w616, "DAO Actions"=DAO_Actions_with_Remove."Set") -> ("error out"=w611:errorcluster)  [unwired: 5 in, 2 out]
              }
            }
          }
          frame "Forces", Default {
            n270 = case shown="True" w625 {
              tunnel: w630 -> [w637 _]
              tunnel: w629 -> [w636 w644]
              tunnel: w628 -> [w634 _]
              tunnel: w627 -> [w633 w645]
              tunnel: [w632 w646] -> w626
              tunnel: w624 -> [_ _]
              tunnel: w623 -> [_ w643]
              tunnel: w622 -> [_ w642]
              tunnel: w621 -> [_ w638]
              frame False {
                n271 = Index Array(array=w637, index=w636) -> (element=w635:refnum<vi>)
                n272 = property class="Clust (strict)"(reference=w635, error in=w633, "Value"=w634) -> (error out=w632:errorcluster)  [unwired: 1 out]
                n273 = One Button Dialog(message="Manual changes not implemented") -> ()  [unwired: 1 in, 1 out]
              }
              frame True {
                n274 = Unbundle By Name(w642) -> ("Table Data 1"=w641:dbl[][])
                n275 = call "Force Table Number 2 Dataset Id.vi"("Table Number"=w644) -> ("Dataset Source"=w649:T4, "Dataset Type"=w648:T5)  [unwired: 3 in]
                n276 = Index Array(array=w641, index (col)=0 ("disabled index (col)")) -> (element=w639:dbl[])  [unwired: 1 in]
                n277 = Bundle By Name(cluster=w643, "Dataset Type"=w648, "Dataset Source"=w649, "Tag"=w638) -> (w647:T3)
                n278 = call "Offsets.vi"("error in (no error)"=w645, "Dataset Trans Id"=w647, "Data In"=w639, "DAO Actions"=DAO_Actions_with_Remove."Set") -> ("error out"=w646:errorcluster)  [unwired: 5 in, 2 out]
              }
            }
          }
        }
        n279 = local read "Cartesian Type"() -> (w562:bool)
        n280 = for {
          tunnel: w564 -> [w586]
          tunnel: w566 -> [w585] mode=indexing
          tunnel: w562 -> [w582]
          tunnel: w563 -> [w584]
          tunnel: w565 -> [w581]
          tunnel: w560 -> [w583]
          shift-right: [w589] -> w568
          shift-left: w567 -> [w591]
          shift-right: [w590] -> w569
          shift-left: w570 -> [w588]
          n281 = Bundle By Name(cluster=w586, "Update Offset Actions"=w585, "Offset Type"=w584, "Coordinate Space"=w581, "Cartesian Type"=w582, "Tag"=w583) -> (w587:T12)
          n282 = Enqueue Element(queue=w591, element=w587, error in (no error)=w588) -> (queue out=w589:refnum<queue>, error out=w590:errorcluster)  [unwired: 1 in, 1 out]
        }
      }
      event Timeout {
        n283 = event-data() -> ()  [unwired: 4 out]
        n284 = local write "Execute"(FALSE ("Calculate")) -> ()
        n285 = local read "Force Offset Tag"() -> (w654:u16)
        n286 = local read "Offset Type"() -> (w653:T8)
        n287 = local read "Coordinate Space"() -> (w652:T7)
        n288 = local read "Cartesian Type"() -> (w651:bool)
        n289 = property on="Force Offset Tag" class="Ring (strict)"() -> ("Strings []"=w655:string[])  [unwired: 2 in, 2 out]
        n290 = Index Array(array=w655, index=w654) -> (element=w663:string)
        n291 = Bundle By Name(cluster=w656, "Update Offset Actions"=Update_Offset_Actions."Update Table" ("element"), "Offset Type"=w653, "Coordinate Space"=w652, "Cartesian Type"=w651, "Tag"=w663) -> (w657:T12)
        n292 = Enqueue Element(queue=w661, element=w657, error in (no error)=w658) -> (queue out=w660:refnum<queue>, error out=w659:errorcluster)  [unwired: 1 in, 1 out]
      }
    }
  }
  "error out" <- w25
  n293 = Compound Arithmetic op=AND(w24, w23) -> (w22:bool)
  n294 = flat-sequence {
    tunnel: w22 -> [w671]
    frame #0 {
      n295 = Not(x=w671) -> (.not. x?=w670:bool)
      n296 = local write "Cancel"(w670) -> ()
      n297 = control-ref of="This VI"() -> (w667:refnum<vi>)
      n298 = local write "Ok"(w670) -> ()
      n299 = property class="VI"(reference=w667) -> ("Front Panel.Open"=w666:bool)  [unwired: 1 in, 2 out]
      n300 = case shown="True" w666 {
        tunnel: w667 -> [_ w672]
        frame False {
        }
        frame True {
          n301 = invoke class="VI" method="FP.Close"(reference=w672) -> ()  [unwired: 2 in, 3 out]
        }
      }
      n302 = call "NoArgumentsLauncher.vi"("Application"=NoPanelAppTypes."Offsets", "Application Launcher Actions"=Launcher_Actions."Stop") -> ()  [unwired: 1 in, 9 out]
    }
  }
